vi "detNbrStepsInProfile.vi"(8 "error in (no error)":errorcluster, 11 "TestMonitor in":refnum<class "TestMonitor.lvclass">) -> (0 "error out":errorcluster, 3 "TestMonitor out":refnum<class "TestMonitor.lvclass">)   [LabVIEW 2013, in "TestMonitor.lvclass"]
uses:
  TestMonitor.lvclass
  TestMonitor.lvclass/TestMonitor.ctl
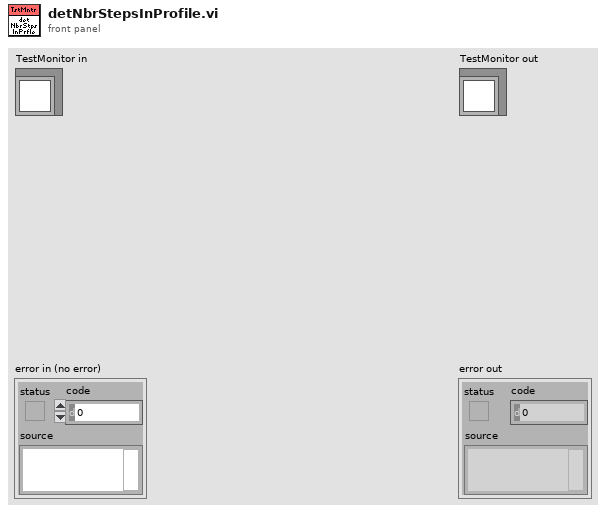
[diagram p1: front panel]
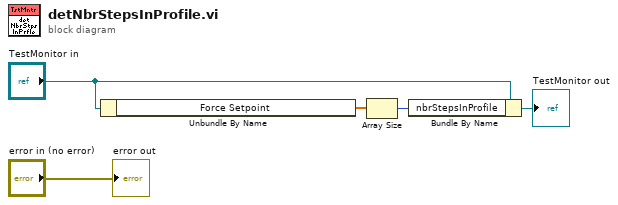
[diagram p0: block diagram]
diagram:
  n1 = Unbundle By Name("TestMonitor in") -> ("Force Setpoint"=w4:dbl[unit][])
  n2 = Array Size(array=w4) -> (size(s)=w3:i32)
  n3 = Bundle By Name(cluster="TestMonitor in", "nbrStepsInProfile"=w3) -> (→"TestMonitor out":refnum<class "TestMonitor.lvclass">)
  "error out" <- "error in (no error)"
